vi "DutyCycleOut Setter.vi"(0 "DeviceReference":T1, 1 "OverrideBrakeDurNeutral":bool, 2 "LimitReverseMotion":bool, 3 "Update Frequency (Hz)":dbl=100.0, 5 "StopSendingOtherRequests":bool=TRUE, 7 "Output":dbl, 9 "EnableFOC":bool=TRUE, 12 "LimitForwardMotion":bool) -> (4 "DeviceReference Out":T1)   [LabVIEW 2023]
doc: "Request a specified motor duty cycle.\nThis control mode will output a proportion of the supplied voltage which is supplied by the user."
uses:
  Users/Cory/Documents/PhoenixPro-LabVIEW-Generation/controls/DeviceReference.ctl
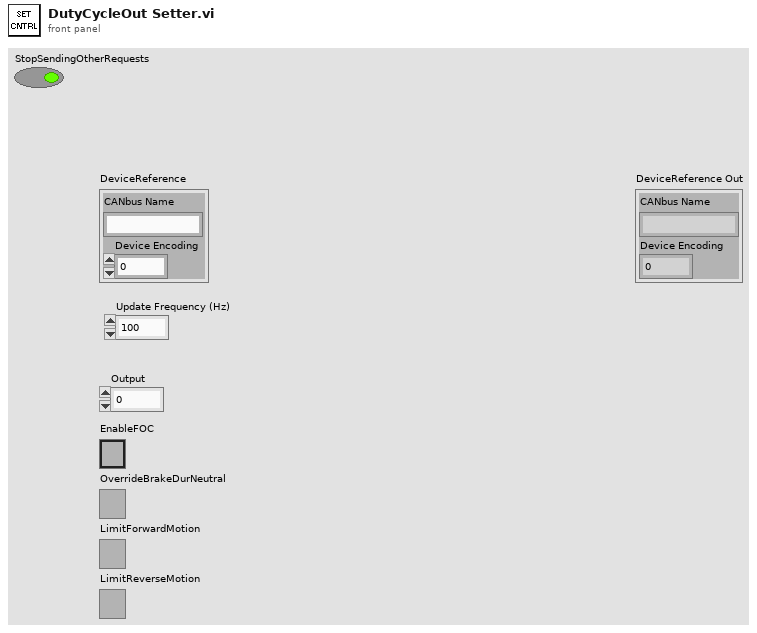
[diagram p1: front panel]
types:
  T1 = typedef "DeviceReference.ctl" = cluster{"CANbus Name":string, "Device Encoding":u32}
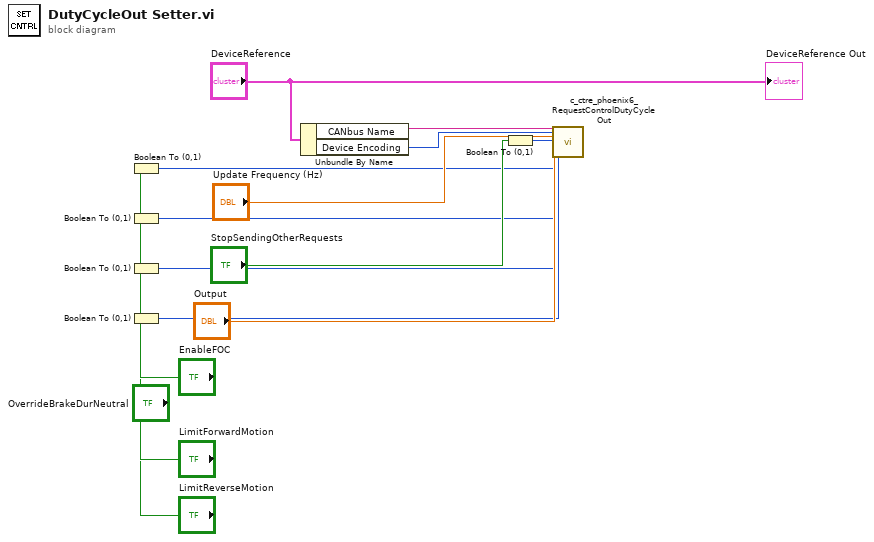
[diagram p0: block diagram]
diagram:
  n1 = Boolean To (0,1)(Boolean="EnableFOC") -> (0, 1=w7:i16)
  n2 = Boolean To (0,1)(Boolean="OverrideBrakeDurNeutral") -> (0, 1=w5:i16)
  n3 = Boolean To (0,1)(Boolean="LimitForwardMotion") -> (0, 1=w3:i16)
  n4 = Boolean To (0,1)(Boolean="LimitReverseMotion") -> (0, 1=w1:i16)
  n5 = Unbundle By Name("DeviceReference") -> ("CANbus Name"=w14:string, "Device Encoding"=w13:u32)
  n6 = Boolean To (0,1)(Boolean="StopSendingOtherRequests") -> (0, 1=w10:i16)
  n7 = call <vilib>:"c_ctre_phoenix6_RequestControlDutyCycleOut.vi"("String"=w14, "Numeric 2"=w13, "Numeric 3"="Update Frequency (Hz)", "Numeric 4"=w10, "Numeric 5"="Output", "Numeric 6"=w7, "Numeric 7"=w5, "Numeric 8"=w3, "Numeric 9"=w1) -> ()  [unwired: 18 in, 1 out]
  "DeviceReference Out" <- "DeviceReference"
